vi "ADC INL_ref_sweep.vi"(8 "error in (no error)":errorcluster, 9 "Sequence parameters":string[][](array[string])=[["Min limit", "Max limit", "Register sheet file", "Register Sheet"], ["", "", "CC2600.xls", "TX_BLE;Trim"], ["Reg write (addr;value)", "Operating frequency [Hz]", "", ""], ["NA", "2.44G", "", ""]], 10 "Run type":i32, 11 "Method parameters":T3={"Dev"={"Do not disturb DUT"=FALSE, "XOSC"=32000000.0, "Board type"="", "EM"="", "Configure tempboard"=TRUE, "Device specific info"=[], "Generic Object"=refnum}, "Method"={"Run type"=1, "Test name"="Current LPM2 4", "Comment"="", "Results folder"="", "AFC"=enum."Off", "Method name"="Current LPM2 4", "Method results"={"Excel brief report"=FALSE, "Spotfire report"=FALSE, "Starfish report"=FALSE}, "Operator"="", "Reference time"=timestamp(0 s since 1904-01-01), "AFC delay"=0.0, "Initialization"=enum."Enabled", "MD5 Sum"="", "HW addon board"=enum."None", "AFC Regsheet"="", "AFC Regfile"=path "", "dummy"=0.0}, "Inst"={"Instr"={"PS1"={"Name"="", "GPIB address"="", "VISA session"=""}, "PS2"={"Name"="", "GPIB address"="", "VISA session"=""}, "TC1"={"Name"="", "GPIB address"="", "VISA session"=""}, "TC2"={"Name"="", "GPIB address"="", "VISA session"=""}, "SA1"={"Name"="", "GPIB address"="", "VISA session"=""}, "SA2"={"Name"="", "GPIB address"="", "VISA session"=""}, "SG1"={"Name"="", "GPIB address"="", "VISA session"=""}, "SG2"={"Name"="", "GPIB address"="", "VISA session"=""}, "SG3"={"Name"="", "GPIB address"="", "VISA session"=""}, "MI1"={"Name"="", "GPIB address"="", "VISA session"=""}, "MI2"={"Name"="", "GPIB address"="", "VISA session"=""}, "SW SA"={"Name"="", "Controller addr"=""}, "SW SG"={"Name"="", "Controller addr"=""}, "MI3"={"Name"="", "GPIB address"="", "VISA session"=""}}, "Switchbox"={"RF Path"=0, "Cal compensation"=enum."TX", "Switchbox gain mode"="", "State"=enum."TX"}, "Instr to control (i.e. SA1)"="Default", "Intrument info string"=""}, "Sequence parameters"=[["Weight", "Min Limit", "Max Limit", "Register Sheet", "", "", "", "", "", "", "", "", ""], ["Vital", "", "1", "LPM2", "", "", "", "", "", "", "", "", ""], ["Resolution", "Reg write (addr;value)", "Chip mode", "Range", "", "", "", "", "", "", "", "", ""], ["u", "NA", "", "auto", "", "", "", "", "", "", "", "", ""]], "Cond"={"Temp logged"=25.0, "VDD1_PS1_6V"=-999.0, "VDD2_PS1_25V"=-999.0, "VDD4_PS2_25V"=-999.0, "VDD3_PS2_6V"=-999.0}, "Meas config"={"X-axis inner loop index"=32000000, "Y-axis outer loop index"=32000000, "X-axis"=[], "Y-axis"=[], "X-axis array req size"=32000000, "Y-axis array req size"=32000000, "Param description"=[], "Use meas clust for reporting"=FALSE, "Parameter index (page)"=0, "X-axis name"="", "Y-axis name"=""}} {"Cond"."VDD3_PS2_6V" format="%.3f"; "Cond"."VDD4_PS2_25V" format="%.3f"; "Cond"."VDD2_PS1_25V" format="%.3f"; "Cond"."VDD1_PS1_6V" format="%.3f"; "Method"."dummy" format="%.1p"; "Method"."AFC delay" format="%.1p"; "Dev"."XOSC" format="%.3p"}) -> (0 "error out":errorcluster, 1 "End method error":T2, 2 "Short Results":string[](array[string])=["0.00", "0.00", "0.00", "0.00"], 3 "Result summary":string[][](array[string])=[["Critical", "Output Power@2405 MHz", "-3", "4", "dBm"], ["Critical", "Output Power@2410 MHz", "-3", "4", "dBm"]])   [LabVIEW 2019]
doc: "[AutoDocStart]Performs crystal accuracy measurements. Measures the offset from ideal frequency. Primarily used for tuning XOSC capacitors and verifying XOSC trims.\n\nSweeping parameters: operating frequency, OSC override value and VDDR level\n\nResults: Offset frequency in ppm[AutoDocEnd]"
uses:
  User Lib/Utilities/Cluster definitions/Method input.ctl
  User Lib/Utilities/Cluster definitions/Device specific info.ctl
  User Lib/Utilities/Controls/Automatic Frequency Compensation types.ctl
  User Lib/Utilities/Controls/Method Reports.ctl
  User Lib/Utilities/Cluster definitions/Method Initialization.ctl
  User Lib/Utilities/Controls/HW addon boards.ctl
  User Lib/Utilities/Cluster definitions/Instr clust.ctl
  User Lib/Utilities/Switchbox control/SwitchBox_State._ENUMctl.ctl
  User Lib/Utilities/Cluster definitions/End method error cluster.ctl
  User Lib/Utilities/Cluster definitions/DUT vdd control.ctl
  User Lib/Utilities/Cluster definitions/DUT VDD4.ctl
  User Lib/Utilities/Cluster definitions/DUT VDD3.ctl
  User Lib/Utilities/Cluster definitions/DUT VDD2.ctl
  User Lib/Utilities/Cluster definitions/DUT VDD1.ctl
  62b45376-0a3e-4237-a030-b0a612edc8e5.vi
  47332434-656c-4693-9234-e05a15154894.vi
  4dd78ca8-5857-4938-84a9-ce08f9b77024.vi
  42f514b6-df04-40b6-a03b-a487344522a2.vi
  9f9df643-cad2-47cb-a2d6-a9993951f146.vi
  b7ff9f93-cf4b-49d2-9220-d5c2ebaf56eb.vi
  d5327cad-c336-4ca6-ac46-e2641e1e3ffd.vi
  0285ada5-cea9-4f7c-8e18-3c0901f4aec6.vi
  6c98f5ed-e302-4408-84f7-1c72ba02b448.vi
  444cb217-8591-421e-8a66-875f56f40be3.vi
  21c70261-1cdc-4561-82c9-de3bd15db41d.vi
  b9949edb-c3cc-4db3-98e4-a09d5f44d9c3.vi
panel:
  in  "Tab Control":T1(tab)
  # "°C"
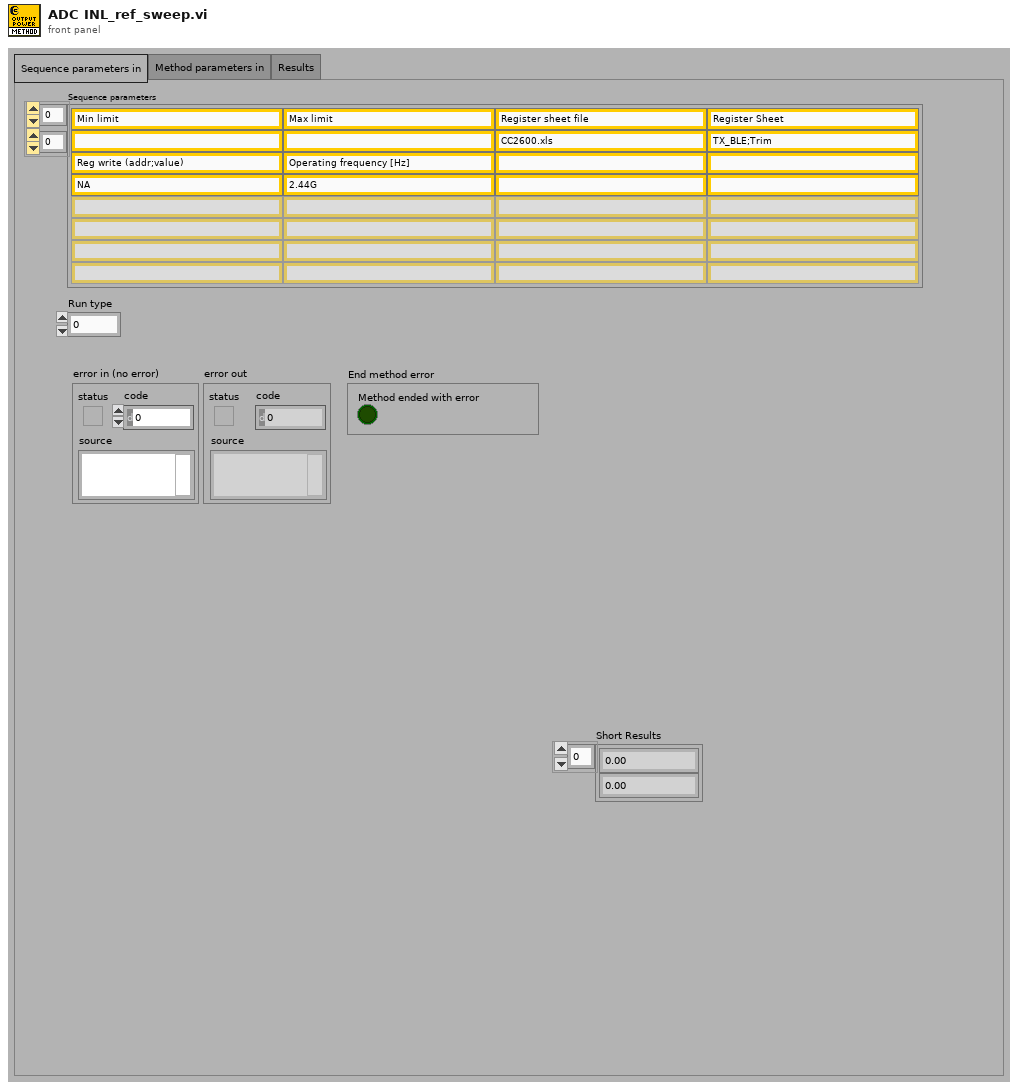
[diagram p1: front panel]
types:
  T1 = enum32{"Sequence parameters in", "Method parameters in", "Results"}
  T2 = typedef "End method error cluster.ctl" = cluster{"Method ended with error":bool}
  T3 = typedef "Method input.ctl" = cluster{"Dev":cluster{"Do not disturb DUT":bool, "XOSC":dbl, "Board type":string, "EM":string, "Configure tempboard":bool, "Device specific info":T4[], "Generic Object":refnum<class>}, "Method":cluster{"Run type":i32, "Test name":string, "Comment":string, "Results folder":string, "AFC":T5, "Method name":string, "Method results":T6, "Operator":string, "Reference time":timestamp, "AFC delay":dbl, "Initialization":T7, "MD5 Sum":string, "HW addon board":T8, "AFC Regsheet":string, "AFC Regfile":path, "dummy":dbl}, "Inst":T9, "Sequence parameters":string[][], "Cond":cluster{"Temp logged":dbl, "VDD1_PS1_6V":dbl, "VDD2_PS1_25V":dbl, "VDD4_PS2_25V":dbl, "VDD3_PS2_6V":dbl}, "Meas config":cluster{"X-axis inner loop index":i32, "Y-axis outer loop index":i32, "X-axis":string[], "Y-axis":string[], "X-axis array req size":i32, "Y-axis array req size":i32, "Param description":string[][], "Use meas clust for reporting":bool, "Parameter index (page)":i32, "X-axis name":string, "Y-axis name":string}}
  T4 = typedef "Device specific info.ctl" = cluster{"EM number":u8, "IP address":string, "Enabled":bool, "Slot no":u8, "RF path":u8, "EM name":string, "Wafer info":string, "AFC frequency ppm":dbl, "Register writes":string[][], "Meas data":string[][][], "Device comment":string}
  T5 = typedef "Automatic Frequency Compensation types.ctl" = enum16{"Off", "Compensate Instrument frequency", "Compensate DUT frequency", "Predictive - Compensate Instrument frequency", "Predictive - Compensate DUT frequency", "Do not skip re-init - Compensate Instrument frequency", "Do not skip re-init - Compensate DUT frequency"}
  T6 = typedef "Method Reports.ctl" = cluster{"Excel brief report":bool, "Spotfire report":bool, "Starfish report":bool}
  T7 = typedef "Method Initialization.ctl" = enum16{"Enabled", "Skip Instr and Device Init", "Enabled with Separate Flash", "Set PS, Device Init and Skip Instr Init", "Skip Device Init"}
  T8 = typedef "HW addon boards.ctl" = enum16{"None", "Current meas 5EM", "Stresstest 10EM"}
  T9 = typedef "Instr clust.ctl" = cluster{"Instr":cluster{"PS1":cluster{"Name":string, "GPIB address":string, "VISA session":refnum<visa-resource-name>}, "PS2":cluster{"Name":string, "GPIB address":string, "VISA session":refnum<visa-resource-name>}, "TC1":cluster{"Name":string, "GPIB address":string, "VISA session":refnum<visa-resource-name>}, "TC2":cluster{"Name":string, "GPIB address":string, "VISA session":refnum<visa-resource-name>}, "SA1":cluster{"Name":string, "GPIB address":string, "VISA session":refnum<visa-resource-name>}, "SA2":cluster{"Name":string, "GPIB address":string, "VISA session":refnum<visa-resource-name>}, "SG1":cluster{"Name":string, "GPIB address":string, "VISA session":refnum<visa-resource-name>}, "SG2":cluster{"Name":string, "GPIB address":string, "VISA session":refnum<visa-resource-name>}, "SG3":cluster{"Name":string, "GPIB address":string, "VISA session":refnum<visa-resource-name>}, "MI1":cluster{"Name":string, "GPIB address":string, "VISA session":refnum<visa-resource-name>}, "MI2":cluster{"Name":string, "GPIB address":string, "VISA session":refnum<visa-resource-name>}, "SW SA":cluster{"Name":string, "Controller addr":string}, "SW SG":cluster{"Name":string, "Controller addr":string}, "MI3":cluster{"Name":string, "GPIB address":string, "VISA session":refnum<visa-resource-name>}}, "Switchbox":cluster{"RF Path":i32, "Cal compensation":enum16{"TX", "RX", "Interferer", "No compensation", "Interferer2"}, "Switchbox gain mode":string, "State":T10}, "Instr to control (i.e. SA1)":string, "Intrument info string":string}
  T10 = typedef "SwitchBox_State._ENUMctl.ctl" = enum16{"TX", "RX", "SP:TX", "SP:RX", "SW:TX", "SW:RX"}
  T11 = typedef "DUT vdd control.ctl" = cluster{"VDD4 config":T12, "VDD3 config":T13, "VDD2 config":T14, "VDD1 config":T15}
  T12 = typedef "DUT VDD4.ctl" = u16
  T13 = typedef "DUT VDD3.ctl" = u16
  T14 = typedef "DUT VDD2.ctl" = u16
  T15 = typedef "DUT VDD1.ctl" = u16
  T16 = enum32{"NI Card Settings", "Memory Read Setting", "DC Capture", "ADC Ramp", "ADC Sine", "SNR", "Cap Calibration"}
  T17 = enum32{"Read from Memory", "Read .dat file", "NI Card Capture", "None"}
  T18 = cluster{"Path to Save plot":path, "Path to Raw Data plot":path}
  T19 = cluster{"Save INL/DNL Plot(Ramp)":bool, "Save SNR Plot":bool, "Save INL/DNL Plot(Sine)":bool, "Save INL/DNL Raw Data(Ramp)":bool, "Save SNR Raw Data":bool, "Save INL/DNL Raw Data(Sine)":bool, "Save DC Raw data":bool, "Save  Raw Data(Sine)":bool}
  T20 = cluster{"Min INL":dbl, "Max INL":dbl, "Min DNL":dbl, "Max DNL":dbl, "INL Range":dbl, "DNL Range":dbl, "Avg Hits/Code":dbl}
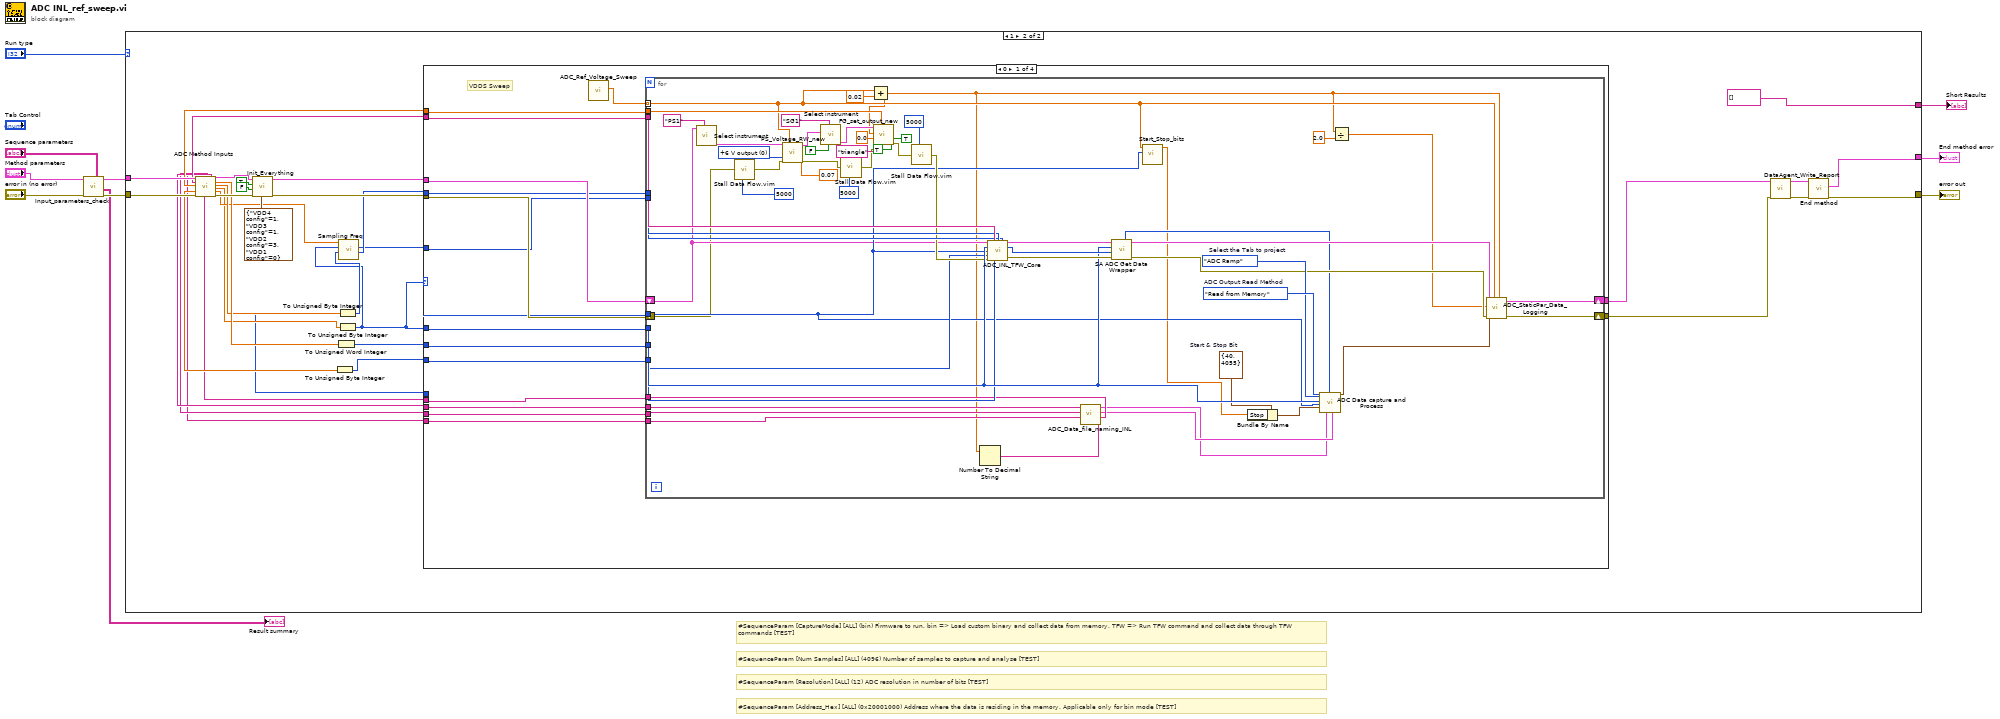
[diagram p0: block diagram]
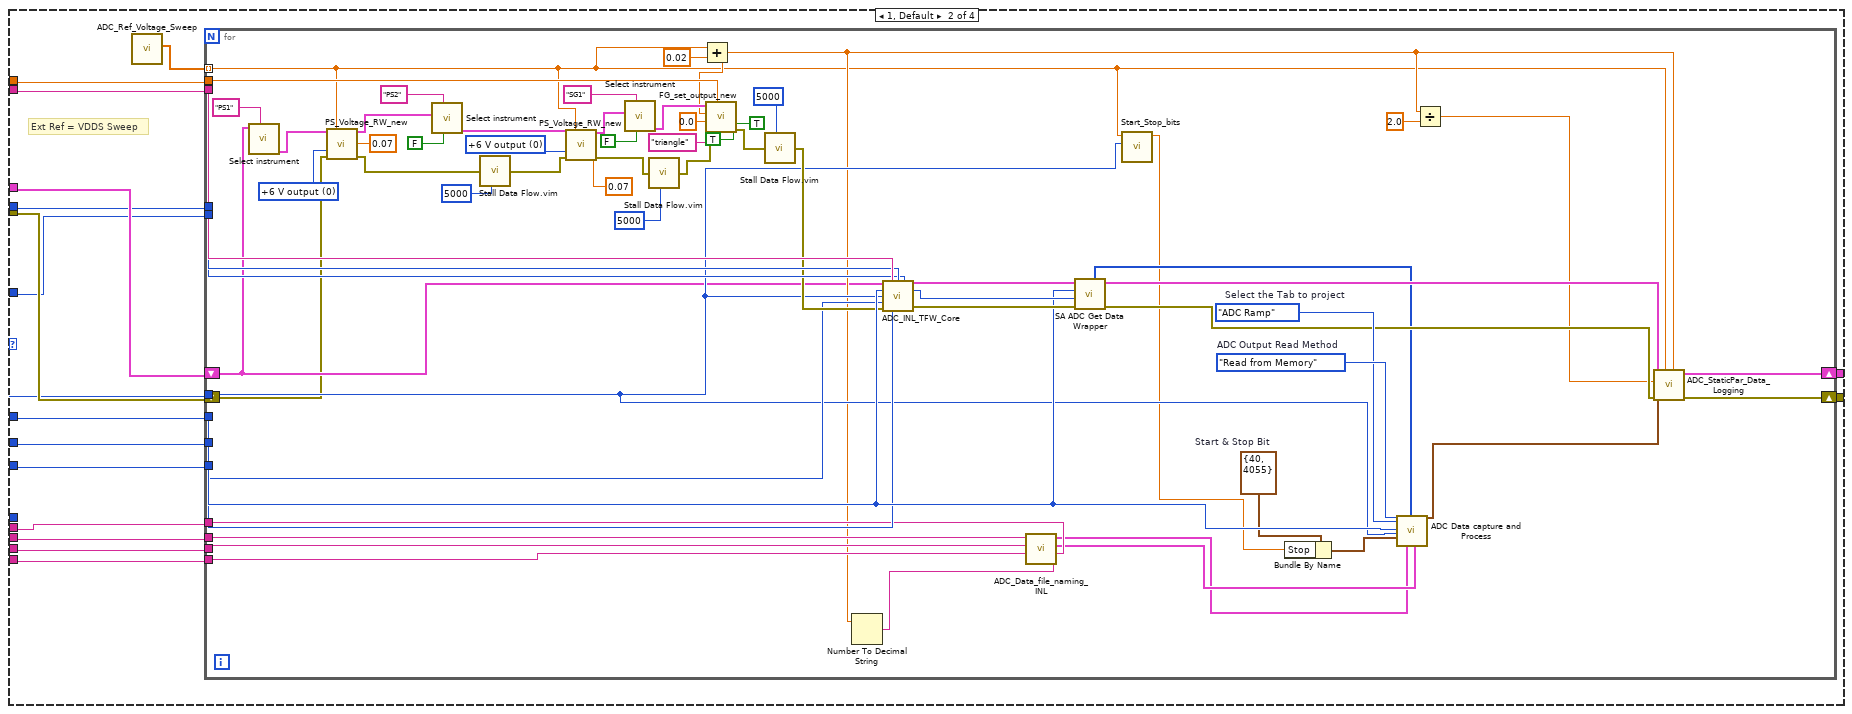
[diagram p3: hidden frame]
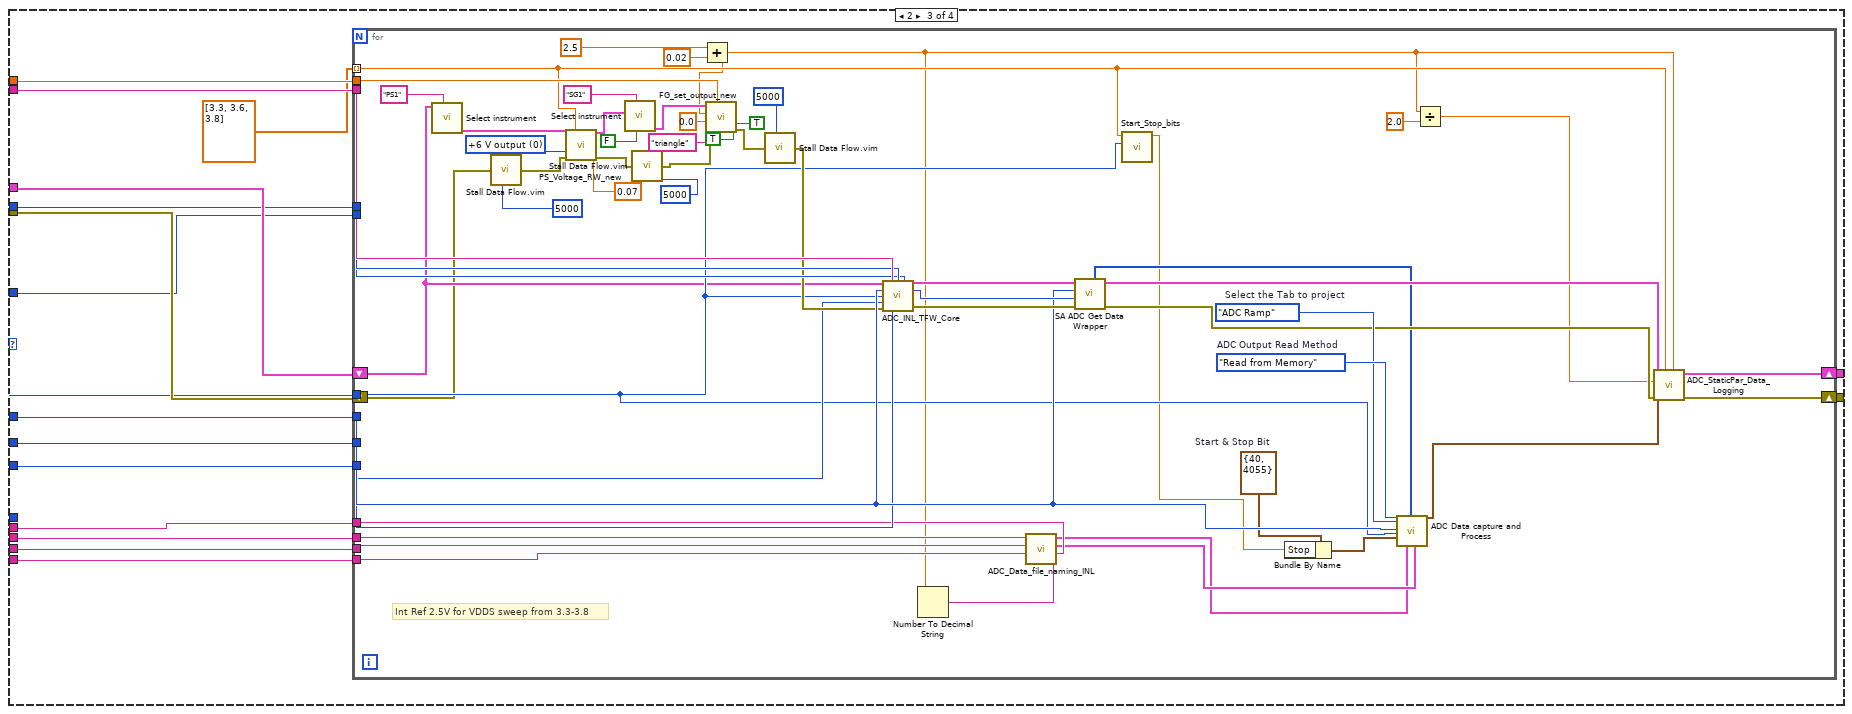
[diagram p4: hidden frame]
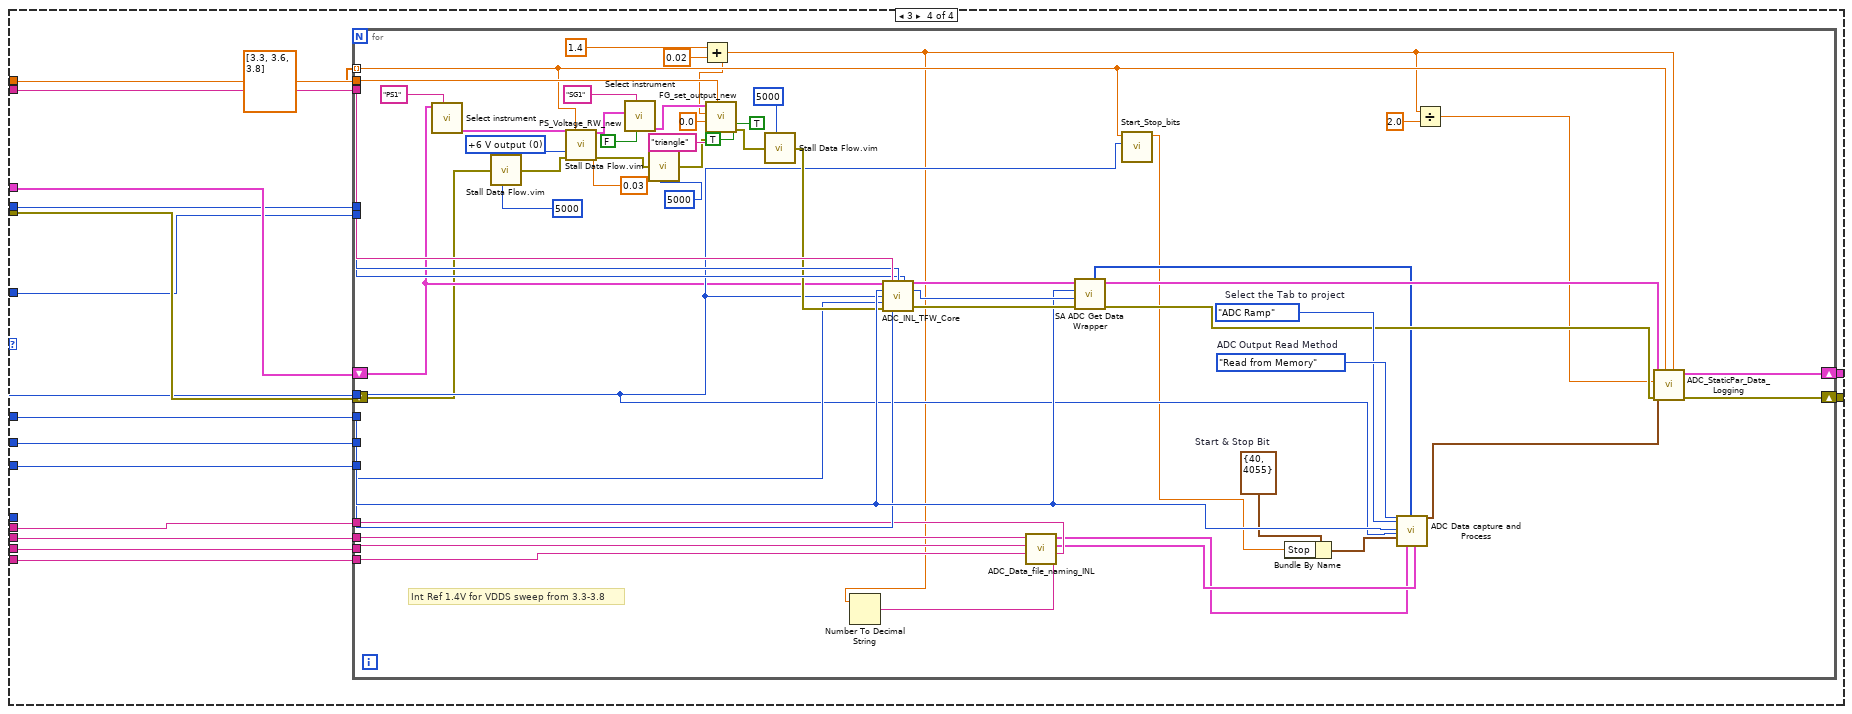
[diagram p5: hidden frame]
diagram:
  # "#SequenceParam [Num Samples] [ALL] (4096) Number of samples to capture and analyse [TEST]"
  # "#SequenceParam [CaptureMode] [ALL] (bin) Firmware to run. bin => Load custom binary and collect data from memory. TFW => Run TFW command and collect data through TFW commands [TEST]"
  # "#SequenceParam [Address_Hex] [ALL] (0x20001000) Address where the data is residing in the memory. Applicable only for bin mode [TEST]"
  # "#SequenceParam [Resolution] [ALL] (12) ADC resolution in number of bits [TEST]"
  n1 = call "Input_parameters_check.vi"("Sequence parameters"="Sequence parameters", "error in"="error in (no error)", "Method cluster in"="Method parameters") -> ("error out"=w9:errorcluster, "Result summary"=→"Result summary":string[][], "Method cluster out"=w5:T3)  [unwired: 6 in]
  n2 = case shown="1" "Run type" {
    tunnel: w9 -> [w11 w33]
    tunnel: [w11 w44] -> w10
    tunnel: w5 -> [_ w34]
    tunnel: [_ w43] -> w4
    tunnel: [_ string[] []] -> w1
    frame 0, Default {
      # "Run type 0 is only for formatting the result summary"
    }
    frame 1 {
      n3 = call "ADC Method Inputs.vi"("Method cluster in"=w34, "error in (no error)"=w33) -> ("Capture Mode"=w21:string, "Signal Freq"=w17:dbl, "ADC Chnl No."=w26:dbl, "Sampling Freq String"=w14:string, "Chnl No. string"=w13:string, "Resolution String"=w15:string, "Voltage Ref String"=w16:string, "Method cluster out"=w31:T3, "Num Samples"=w30:dbl, "Resolution"=w29:dbl, "Voltage Ref"=w27:dbl, "Sampling Freq"=w28:dbl, "error out"=w32:errorcluster)  [unwired: 3 in, 2 out]
      n4 = call "Init_Everything.vi"("VDD config"=T11 {"VDD4 config"=1, "VDD3 config"=1, "VDD2 config"=3, "VDD1 config"=0}, "error in"=w32, "Support current measurement?"=FALSE, "Override VDD Config"=TRUE, "Method cluster In"=w31) -> ("error out"=w25:errorcluster, "Method cluster out"=w12:T3)  [unwired: 3 in, 2 out]
      n5 = To Unsigned Byte Integer(number=w26) -> (unsigned 8bit integer=w22:u8)
      n6 = To Unsigned Word Integer(number=w30) -> (unsigned 16bit integer=w24:u16)
      n7 = To Unsigned Byte Integer(number=w29) -> (unsigned 8bit integer=w23:u8)
      n8 = To Unsigned Byte Integer(number=w27) -> (unsigned 8bit integer=w18:u8)
      n9 = call "Sampling Freq.vi"("Resolution"=w23, "Voltage Ref"=w18, "Sampling Freq"=w28) -> ("LGPT Count"=w20:u16, "SCOMP"=w19:u16)  [unwired: 7 in]
      n10 = case shown="0" w18 {
        tunnel: [w61 w134 w214 w288] -> w38
        tunnel: [w60 w133 w213 w287] -> w37
        tunnel: w12 -> [w59 w132 w212 w286]
        tunnel: w25 -> [w58 w131 w211 w285]
        tunnel: w24 -> [w57 w130 w210 w284]
        tunnel: w23 -> [w56 w129 w209 w283]
        tunnel: w18 -> [w55 w128 w208 w282]
        tunnel: w22 -> [w54 w127 w207 w281]
        tunnel: w21 -> [w53 w126 w206 w280]
        tunnel: w20 -> [w52 w125 w205 w279]
        tunnel: w19 -> [w51 w124 w204 w278]
        tunnel: w17 -> [w49 w122 w203 w277]
        tunnel: w16 -> [w48 w121 w202 w276]
        tunnel: w15 -> [w47 w120 w201 w275]
        tunnel: w14 -> [w46 w119 w200 w274]
        tunnel: w13 -> [w45 w118 w199 w273]
        frame 0 {
          # "VDDS Sweep"
          n11 = call "ADC_Ref_Voltage_Sweep.vi"() -> ("Ref voltage sweep"=w50:dbl[])  [unwired: 11 in]
          n12 = for {
            tunnel: w57 -> [w106]
            tunnel: w56 -> [w84]
            tunnel: w55 -> [w85]
            tunnel: w54 -> [w105]
            tunnel: w53 -> [w104]
            tunnel: w52 -> [w103]
            tunnel: w51 -> [w102]
            shift-right: [w112] -> w61
            shift-left: w59 -> [w79]
            shift-right: [w111] -> w60
            shift-left: w58 -> [w73]
            tunnel: w50 -> [w68] mode=indexing
            tunnel: w49 -> [w94]
            tunnel: w48 -> [w91]
            tunnel: w47 -> [w90]
            tunnel: w46 -> [w89]
            tunnel: w45 -> [w88]
            w80 = u16 0 items=["+6 V output", "+25 V output", "-25 V output", "ALL TERM"] ("Output Terminals")
            w83 = cluster{"Start":i32, "Stop":i32} {"Start"=40, "Stop"=4055}  # Start & Stop Bit
            w116 = T16."ADC Ramp"  # Select the Tab to project
            w117 = T17."Read from Memory"  # ADC Output Read Method
            n13 = call "Select instrument.vi"("Instr.Instr to control (i.e. SA1)"="PS1", "Method cluster in"=w79) -> ("Instr out"=w78:T9)  [unwired: 7 in, 2 out]
            n14 = call "Stall Data Flow.vim"("value in"=w73, "milliseconds to wait"=u32 5000) -> ("value out"=w74:errorcluster)  [unwired: 1 out]
            n15 = call "PS_Voltage_RW_new.vi"("InstrCluster in"=w78, "Set Voltage"=w68, "Current(0)"=0.07, "Output Terminals"=w80, "error in (no error)"=w74) -> ("InstrCluster out"=w77:T9, "error out"=w64:errorcluster)  [unwired: 8 in, 1 out]
            n16 = call "Select instrument.vi"("Method cluster (T) / Instr cluster (F)"=FALSE, "Instr.Instr to control (i.e. SA1)"="SG1", "Instr in"=w77) -> ("Instr out"=w101:T9)  [unwired: 6 in, 2 out]
            n17 = call "Stall Data Flow.vim"("value in"=w64, "milliseconds to wait"=u32 5000) -> ("value out"=w63:errorcluster)  [unwired: 1 out]
            n18 = Add(x=w68, y=0.02) -> (x+y=w66:dbl)
            n19 = call "FG_set_output_new.vi"("High impedance (T)"=TRUE, "Enable Output?"=TRUE, "Function (DC, Sine, Square, Triangle, Ramp up, Ramp down, Pulse)"="triangle", "Frequency [Hz]"=w94, "error in"=w63, "Low voltage"=0.0, "High voltage (or DC)"=w66, "InstrCluster in"=w101) -> ("error out"=w99:errorcluster)  [unwired: 2 in, 1 out]
            n20 = call "Stall Data Flow.vim"("value in"=w99, "milliseconds to wait"=u32 5000) -> ("value out"=w98:errorcluster)  [unwired: 1 out]
            n21 = Number To Decimal String(number=w66) -> (decimal integer string=w67:string)  [unwired: 1 in]
            n22 = call "ADC_INL_TFW_Core.vi"("Method cluster in"=w79, "Capture Mode"=w104, "LGPT Count"=w103, "SCOMP"=w102, "No. Samples"=w106, "Resolution"=w84, "Voltage Ref"=w85, "error in"=w98, "ADC Chnl No."=w105) -> ("Method cluster out"=w108:T3, "ResPar[0] Data Address"=w107:u32, "error out"=w109:errorcluster)  [unwired: 3 in, 1 out]
            n23 = call "ADC_Data_file_naming_INL.vi"("Amplitude (Vpp)"=w67, "ADC Chn. No"=w88, "Sampling Freq String"=w89, "Resolution String"=w90, "Voltage Ref String"=w91) -> ("path to save"=w87:T18, "Save data"=w86:T19)  [unwired: 5 in]
            n24 = call "SA ADC Get Data Wrapper.vi"("error in"=w109, "Data Address"=w107, "Num Samples"=w106, "Method cluster in"=w108) -> ("error out"=w115:errorcluster, "output cluster"=w114:T3, "ADC samples"=w113:u32[])  [unwired: 2 in, 3 out]
            n25 = call "Start_Stop_bits.vi"("Resolution"=w84, "Input Amplitude"=w68) -> ("Stop Bit"=w81:dbl)  [unwired: 9 in]
            n26 = Bundle By Name(cluster=w83, "Stop"=w81) -> (w82:cluster{"Start":i32, "Stop":i32})
            n27 = call "ADC Data capture and Process.vi"("ADC Output Read Method"=w117, "Select the Tab to project"=w116, "No.of samples"=w106, "Resolution"=w84, "Start & Stop Bit"=w82, "Save data"=w86, "Input Waveform"=w113, "path to save"=w87) -> ("Static Parameters (Ramp)"=w110:T20)  [unwired: 14 in, 5 out]
            n28 = Divide(x=w66, y=2.0) -> (x/y=w70:dbl)
            n29 = call "ADC_StaticPar_Data_Logging.vi"("Offset (V)"=w70, "Amplitude (Vpp)"=w66, "Ref Voltage"=w68, "error in (no error)"=w115, "Static Parameters (Ramp)"=w110, "output cluster"=w114) -> ("error out"=w111:errorcluster, "Method cluster out"=w112:T3)  [unwired: 4 in]
          }
        }
        frame 1, Default {
          # "Ext Ref = VDDS Sweep"
          n30 = call "ADC_Ref_Voltage_Sweep.vi"() -> ("Ref voltage sweep"=w123:dbl[])  [unwired: 11 in]
          n31 = for {
            tunnel: w130 -> [w186]
            tunnel: w129 -> [w164]
            tunnel: w128 -> [w165]
            tunnel: w127 -> [w185]
            tunnel: w126 -> [w184]
            tunnel: w125 -> [w183]
            tunnel: w124 -> [w182]
            shift-right: [w192] -> w134
            shift-left: w132 -> [w148]
            shift-right: [w191] -> w133
            shift-left: w131 -> [w145]
            tunnel: w123 -> [w140] mode=indexing
            tunnel: w122 -> [w174]
            tunnel: w121 -> [w171]
            tunnel: w120 -> [w170]
            tunnel: w119 -> [w169]
            tunnel: w118 -> [w168]
            w139 = u16 0 items=["+6 V output", "+25 V output", "-25 V output", "ALL TERM"] ("Output Terminals")
            w160 = u16 0 items=["+6 V output", "+25 V output", "-25 V output", "ALL TERM"] ("Output Terminals")
            w163 = cluster{"Start":i32, "Stop":i32} {"Start"=40, "Stop"=4055}  # Start & Stop Bit
            w196 = T16."ADC Ramp"  # Select the Tab to project
            w197 = T17."Read from Memory"  # ADC Output Read Method
            n32 = call "Select instrument.vi"("Instr.Instr to control (i.e. SA1)"="PS1", "Method cluster in"=w148) -> ("Instr out"=w146:T9)  [unwired: 7 in, 2 out]
            n33 = call "PS_Voltage_RW_new.vi"("InstrCluster in"=w146, "Set Voltage"=w140, "Current(0)"=0.07, "Output Terminals"=w139, "error in (no error)"=w145) -> ("InstrCluster out"=w142:T9, "error out"=w144:errorcluster)  [unwired: 8 in, 1 out]
            n34 = call "Select instrument.vi"("Method cluster (T) / Instr cluster (F)"=FALSE, "Instr.Instr to control (i.e. SA1)"="PS2", "Instr in"=w142) -> ("Instr out"=w159:T9)  [unwired: 6 in, 2 out]
            n35 = call "Stall Data Flow.vim"("value in"=w144, "milliseconds to wait"=u32 5000) -> ("value out"=w141:errorcluster)  [unwired: 1 out]
            n36 = call "PS_Voltage_RW_new.vi"("InstrCluster in"=w159, "Set Voltage"=w140, "Current(0)"=0.07, "Output Terminals"=w160, "error in (no error)"=w141) -> ("InstrCluster out"=w158:T9, "error out"=w137:errorcluster)  [unwired: 8 in, 1 out]
            n37 = call "Select instrument.vi"("Method cluster (T) / Instr cluster (F)"=FALSE, "Instr.Instr to control (i.e. SA1)"="SG1", "Instr in"=w158) -> ("Instr out"=w181:T9)  [unwired: 6 in, 2 out]
            n38 = call "Stall Data Flow.vim"("value in"=w137, "milliseconds to wait"=u32 5000) -> ("value out"=w136:errorcluster)  [unwired: 1 out]
            n39 = Add(x=w140, y=0.02) -> (x+y=w151:dbl)
            n40 = call "FG_set_output_new.vi"("High impedance (T)"=TRUE, "Enable Output?"=TRUE, "Function (DC, Sine, Square, Triangle, Ramp up, Ramp down, Pulse)"="triangle", "Frequency [Hz]"=w174, "error in"=w136, "Low voltage"=0.0, "High voltage (or DC)"=w151, "InstrCluster in"=w181) -> ("error out"=w179:errorcluster)  [unwired: 2 in, 1 out]
            n41 = call "Stall Data Flow.vim"("value in"=w179, "milliseconds to wait"=u32 5000) -> ("value out"=w178:errorcluster)  [unwired: 1 out]
            n42 = Number To Decimal String(number=w151) -> (decimal integer string=w152:string)  [unwired: 1 in]
            n43 = call "ADC_INL_TFW_Core.vi"("Method cluster in"=w148, "Capture Mode"=w184, "LGPT Count"=w183, "SCOMP"=w182, "No. Samples"=w186, "Resolution"=w164, "Voltage Ref"=w165, "error in"=w178, "ADC Chnl No."=w185) -> ("Method cluster out"=w188:T3, "ResPar[0] Data Address"=w187:u32, "error out"=w189:errorcluster)  [unwired: 3 in, 1 out]
            n44 = call "ADC_Data_file_naming_INL.vi"("Amplitude (Vpp)"=w152, "ADC Chn. No"=w168, "Sampling Freq String"=w169, "Resolution String"=w170, "Voltage Ref String"=w171) -> ("path to save"=w167:T18, "Save data"=w166:T19)  [unwired: 5 in]
            n45 = call "SA ADC Get Data Wrapper.vi"("error in"=w189, "Data Address"=w187, "Num Samples"=w186, "Method cluster in"=w188) -> ("error out"=w195:errorcluster, "output cluster"=w194:T3, "ADC samples"=w193:u32[])  [unwired: 2 in, 3 out]
            n46 = call "Start_Stop_bits.vi"("Resolution"=w164, "Input Amplitude"=w140) -> ("Stop Bit"=w161:dbl)  [unwired: 9 in]
            n47 = Bundle By Name(cluster=w163, "Stop"=w161) -> (w162:cluster{"Start":i32, "Stop":i32})
            n48 = call "ADC Data capture and Process.vi"("ADC Output Read Method"=w197, "Select the Tab to project"=w196, "No.of samples"=w186, "Resolution"=w164, "Start & Stop Bit"=w162, "Save data"=w166, "Input Waveform"=w193, "path to save"=w167) -> ("Static Parameters (Ramp)"=w190:T20)  [unwired: 14 in, 5 out]
            n49 = Divide(x=w151, y=2.0) -> (x/y=w154:dbl)
            n50 = call "ADC_StaticPar_Data_Logging.vi"("Offset (V)"=w154, "Amplitude (Vpp)"=w151, "Ref Voltage"=w140, "error in (no error)"=w195, "Static Parameters (Ramp)"=w190, "output cluster"=w194) -> ("error out"=w191:errorcluster, "Method cluster out"=w192:T3)  [unwired: 4 in]
          }
        }
        frame 2 {
          n51 = for {
            tunnel: w210 -> [w260]
            tunnel: w209 -> [w238]
            tunnel: w208 -> [w239]
            tunnel: w207 -> [w259]
            tunnel: w206 -> [w258]
            tunnel: w205 -> [w257]
            tunnel: w204 -> [w256]
            shift-right: [w266] -> w214
            shift-left: w212 -> [w233]
            shift-right: [w265] -> w213
            shift-left: w211 -> [w227]
            tunnel: dbl[] [3.3, 3.6, 3.8] -> [w222] mode=indexing
            tunnel: w203 -> [w248]
            tunnel: w202 -> [w245]
            tunnel: w201 -> [w244]
            tunnel: w200 -> [w243]
            tunnel: w199 -> [w242]
            w234 = u16 0 items=["+6 V output", "+25 V output", "-25 V output", "ALL TERM"] ("Output Terminals")
            w237 = cluster{"Start":i32, "Stop":i32} {"Start"=40, "Stop"=4055}  # Start & Stop Bit
            w270 = T16."ADC Ramp"  # Select the Tab to project
            w271 = T17."Read from Memory"  # ADC Output Read Method
            # "Int Ref 2.5V for VDDS sweep from 3.3-3.8"
            n52 = call "Select instrument.vi"("Instr.Instr to control (i.e. SA1)"="PS1", "Method cluster in"=w233) -> ("Instr out"=w232:T9)  [unwired: 7 in, 2 out]
            n53 = call "Stall Data Flow.vim"("value in"=w227, "milliseconds to wait"=u32 5000) -> ("value out"=w228:errorcluster)  [unwired: 1 out]
            n54 = call "PS_Voltage_RW_new.vi"("InstrCluster in"=w232, "Set Voltage"=w222, "Current(0)"=0.07, "Output Terminals"=w234, "error in (no error)"=w228) -> ("InstrCluster out"=w231:T9, "error out"=w217:errorcluster)  [unwired: 8 in, 1 out]
            n55 = call "Select instrument.vi"("Method cluster (T) / Instr cluster (F)"=FALSE, "Instr.Instr to control (i.e. SA1)"="SG1", "Instr in"=w231) -> ("Instr out"=w255:T9)  [unwired: 6 in, 2 out]
            n56 = call "Stall Data Flow.vim"("value in"=w217, "milliseconds to wait"=u32 5000) -> ("value out"=w216:errorcluster)  [unwired: 1 out]
            n57 = Add(x=2.5, y=0.02) -> (x+y=w219:dbl)
            n58 = call "FG_set_output_new.vi"("High impedance (T)"=TRUE, "Enable Output?"=TRUE, "Function (DC, Sine, Square, Triangle, Ramp up, Ramp down, Pulse)"="triangle", "Frequency [Hz]"=w248, "error in"=w216, "Low voltage"=0.0, "High voltage (or DC)"=w219, "InstrCluster in"=w255) -> ("error out"=w253:errorcluster)  [unwired: 2 in, 1 out]
            n59 = call "Stall Data Flow.vim"("value in"=w253, "milliseconds to wait"=u32 5000) -> ("value out"=w252:errorcluster)  [unwired: 1 out]
            n60 = call "ADC_INL_TFW_Core.vi"("Method cluster in"=w233, "Capture Mode"=w258, "LGPT Count"=w257, "SCOMP"=w256, "No. Samples"=w260, "Resolution"=w238, "Voltage Ref"=w239, "error in"=w252, "ADC Chnl No."=w259) -> ("Method cluster out"=w262:T3, "ResPar[0] Data Address"=w261:u32, "error out"=w263:errorcluster)  [unwired: 3 in, 1 out]
            n61 = Number To Decimal String(number=w219) -> (decimal integer string=w220:string)  [unwired: 1 in]
            n62 = call "ADC_Data_file_naming_INL.vi"("Amplitude (Vpp)"=w220, "ADC Chn. No"=w242, "Sampling Freq String"=w243, "Resolution String"=w244, "Voltage Ref String"=w245) -> ("path to save"=w241:T18, "Save data"=w240:T19)  [unwired: 5 in]
            n63 = call "SA ADC Get Data Wrapper.vi"("error in"=w263, "Data Address"=w261, "Num Samples"=w260, "Method cluster in"=w262) -> ("error out"=w269:errorcluster, "output cluster"=w268:T3, "ADC samples"=w267:u32[])  [unwired: 2 in, 3 out]
            n64 = call "Start_Stop_bits.vi"("Resolution"=w238, "Input Amplitude"=w222) -> ("Stop Bit"=w235:dbl)  [unwired: 9 in]
            n65 = Bundle By Name(cluster=w237, "Stop"=w235) -> (w236:cluster{"Start":i32, "Stop":i32})
            n66 = call "ADC Data capture and Process.vi"("ADC Output Read Method"=w271, "Select the Tab to project"=w270, "No.of samples"=w260, "Resolution"=w238, "Start & Stop Bit"=w236, "Save data"=w240, "Input Waveform"=w267, "path to save"=w241) -> ("Static Parameters (Ramp)"=w264:T20)  [unwired: 14 in, 5 out]
            n67 = Divide(x=w219, y=2.0) -> (x/y=w224:dbl)
            n68 = call "ADC_StaticPar_Data_Logging.vi"("Offset (V)"=w224, "Amplitude (Vpp)"=w219, "Ref Voltage"=w222, "error in (no error)"=w269, "Static Parameters (Ramp)"=w264, "output cluster"=w268) -> ("error out"=w265:errorcluster, "Method cluster out"=w266:T3)  [unwired: 4 in]
          }
        }
        frame 3 {
          n69 = for {
            tunnel: w284 -> [w334]
            tunnel: w283 -> [w312]
            tunnel: w282 -> [w313]
            tunnel: w281 -> [w333]
            tunnel: w280 -> [w332]
            tunnel: w279 -> [w331]
            tunnel: w278 -> [w330]
            shift-right: [w340] -> w288
            shift-left: w286 -> [w307]
            shift-right: [w339] -> w287
            shift-left: w285 -> [w301]
            tunnel: dbl[] [3.3, 3.6, 3.8] -> [w296] mode=indexing
            tunnel: w277 -> [w322]
            tunnel: w276 -> [w319]
            tunnel: w275 -> [w318]
            tunnel: w274 -> [w317]
            tunnel: w273 -> [w316]
            w308 = u16 0 items=["+6 V output", "+25 V output", "-25 V output", "ALL TERM"] ("Output Terminals")
            w311 = cluster{"Start":i32, "Stop":i32} {"Start"=40, "Stop"=4055}  # Start & Stop Bit
            w344 = T16."ADC Ramp"  # Select the Tab to project
            w345 = T17."Read from Memory"  # ADC Output Read Method
            # "Int Ref 1.4V for VDDS sweep from 3.3-3.8"
            n70 = call "Select instrument.vi"("Instr.Instr to control (i.e. SA1)"="PS1", "Method cluster in"=w307) -> ("Instr out"=w306:T9)  [unwired: 7 in, 2 out]
            n71 = call "Stall Data Flow.vim"("value in"=w301, "milliseconds to wait"=u32 5000) -> ("value out"=w302:errorcluster)  [unwired: 1 out]
            n72 = call "PS_Voltage_RW_new.vi"("InstrCluster in"=w306, "Set Voltage"=w296, "Current(0)"=0.03, "Output Terminals"=w308, "error in (no error)"=w302) -> ("InstrCluster out"=w305:T9, "error out"=w291:errorcluster)  [unwired: 8 in, 1 out]
            n73 = call "Select instrument.vi"("Method cluster (T) / Instr cluster (F)"=FALSE, "Instr.Instr to control (i.e. SA1)"="SG1", "Instr in"=w305) -> ("Instr out"=w329:T9)  [unwired: 6 in, 2 out]
            n74 = call "Stall Data Flow.vim"("value in"=w291, "milliseconds to wait"=u32 5000) -> ("value out"=w290:errorcluster)  [unwired: 1 out]
            n75 = Add(x=1.4, y=0.02) -> (x+y=w293:dbl)
            n76 = call "FG_set_output_new.vi"("High impedance (T)"=TRUE, "Enable Output?"=TRUE, "Function (DC, Sine, Square, Triangle, Ramp up, Ramp down, Pulse)"="triangle", "Frequency [Hz]"=w322, "error in"=w290, "Low voltage"=0.0, "High voltage (or DC)"=w293, "InstrCluster in"=w329) -> ("error out"=w327:errorcluster)  [unwired: 2 in, 1 out]
            n77 = call "Stall Data Flow.vim"("value in"=w327, "milliseconds to wait"=u32 5000) -> ("value out"=w326:errorcluster)  [unwired: 1 out]
            n78 = Number To Decimal String(number=w293) -> (decimal integer string=w294:string)  [unwired: 1 in]
            n79 = call "ADC_INL_TFW_Core.vi"("Method cluster in"=w307, "Capture Mode"=w332, "LGPT Count"=w331, "SCOMP"=w330, "No. Samples"=w334, "Resolution"=w312, "Voltage Ref"=w313, "error in"=w326, "ADC Chnl No."=w333) -> ("Method cluster out"=w336:T3, "ResPar[0] Data Address"=w335:u32, "error out"=w337:errorcluster)  [unwired: 3 in, 1 out]
            n80 = call "ADC_Data_file_naming_INL.vi"("Amplitude (Vpp)"=w294, "ADC Chn. No"=w316, "Sampling Freq String"=w317, "Resolution String"=w318, "Voltage Ref String"=w319) -> ("path to save"=w315:T18, "Save data"=w314:T19)  [unwired: 5 in]
            n81 = call "SA ADC Get Data Wrapper.vi"("error in"=w337, "Data Address"=w335, "Num Samples"=w334, "Method cluster in"=w336) -> ("error out"=w343:errorcluster, "output cluster"=w342:T3, "ADC samples"=w341:u32[])  [unwired: 2 in, 3 out]
            n82 = call "Start_Stop_bits.vi"("Resolution"=w312, "Input Amplitude"=w296) -> ("Stop Bit"=w309:dbl)  [unwired: 9 in]
            n83 = Bundle By Name(cluster=w311, "Stop"=w309) -> (w310:cluster{"Start":i32, "Stop":i32})
            n84 = call "ADC Data capture and Process.vi"("ADC Output Read Method"=w345, "Select the Tab to project"=w344, "No.of samples"=w334, "Resolution"=w312, "Start & Stop Bit"=w310, "Save data"=w314, "Input Waveform"=w341, "path to save"=w315) -> ("Static Parameters (Ramp)"=w338:T20)  [unwired: 14 in, 5 out]
            n85 = Divide(x=w293, y=2.0) -> (x/y=w298:dbl)
            n86 = call "ADC_StaticPar_Data_Logging.vi"("Offset (V)"=w298, "Amplitude (Vpp)"=w293, "Ref Voltage"=w296, "error in (no error)"=w343, "Static Parameters (Ramp)"=w338, "output cluster"=w342) -> ("error out"=w339:errorcluster, "Method cluster out"=w340:T3)  [unwired: 4 in]
          }
        }
      }
      n87 = call "DataAgent_Write_Report.vi"("error in (no error)"=w37, "Method cluster in"=w38) -> ("error out"=w41:errorcluster, "Method cluster out"=w40:T3)  [unwired: 8 in]
      n88 = call "End method.vi"("error in"=w41, "Method cluster in"=w40) -> ("error out"=w44:errorcluster, "End method error"=w43:T2)  [unwired: 7 in, 1 out]
    }
  }
  "error out" <- w10
  "End method error" <- w4
  "Short Results" <- w1
